vi "GetKeyValue_Boolean.vi"(6 "default value":bool, 9 "key":string, 10 "key value pairs":T1[](array[typedef])) -> (1 "value":bool, 2 "key value pairs out":T1[](array[typedef]), 5 "found":bool)   [LabVIEW 2017, in "PropertyHelpers.lvlib"]
doc: "Returns the Boolean value of a particular key in an array of key-value pairs. Use this VI to get properties from the contents of configuration JSON files that the Global Configuration VIs return."
uses:
  <vilib>/addons/InsightCM/Utilities/PropertyHelpers/PropertyHelpers.lvlib
  <vilib>/addons/InsightCM/MessageBus/Base/controls/KeyValuePair.ctl
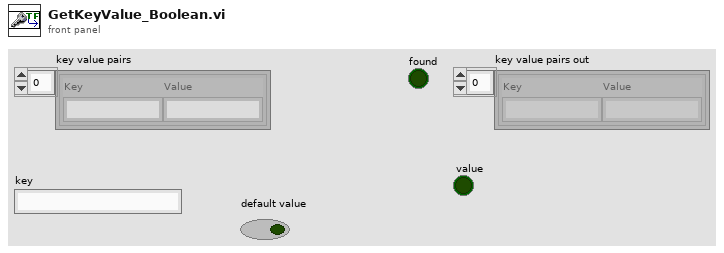
[diagram p1: front panel]
types:
  T1 = typedef "KeyValuePair.ctl" = cluster{"Key":string, "Value":string}
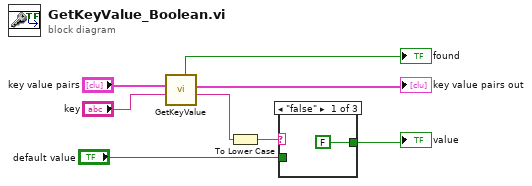
[diagram p0: block diagram]
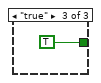
[diagram p3: hidden frame]
diagram:
  n1 = call <vilib>:"GetKeyValue.vi"("key"="key", "key value pairs"="key value pairs") -> ("value"=w5:string, "key value pairs out"=→"key value pairs out":T1[], "found"=→"found":bool)  [unwired: 7 in]
  n2 = To Lower Case(string=w5) -> (all lower case string=w7:string)
  n3 = case shown="\"false\"" w7 {
    tunnel: [FALSE w10 TRUE] -> w6
    tunnel: "default value" -> [_ w10 _]
    frame "false" {
    }
    frame Default {
    }
    frame "true" {
    }
  }
  "value" <- w6
